vi "APDM Hardware.vi"(7 "Gyro Channel In":T3) -> (2 "GPD Message Channel":T2, 3 "Gyro Status Channel":T4)   [LabVIEW 2019]
uses:
  <extravilib>/ChannelInstances/Messenger-t'Gyro Status Message.ctl'/))Channel.ctl
  Lee Lab/CP FES Walking 2018/Code/Working/LabVIEW/Controls/Messages/Gyro Status Message.ctl
  Lee Lab/CP FES Walking 2018/Code/Working/LabVIEW/Controls/States/Gyro Status States.ctl
  <extravilib>/ChannelInstances/Messenger-t'Acquisition Message.ctl'/))Channel.ctl
  Lee Lab/CP FES Walking 2018/Code/Working/LabVIEW/Controls/Messages/Acquisition Message.ctl
  Lee Lab/CP FES Walking 2018/Code/Working/LabVIEW/Controls/States/Acquisition State.ctl
  <extravilib>/ChannelInstances/Messenger-t'GPD Message.ctl'/))Channel.ctl
  Lee Lab/CP FES Walking 2018/Code/Working/LabVIEW/Controls/Messages/GPD Message.ctl
  Lee Lab/CP FES Walking 2018/Code/Working/LabVIEW/Controls/States/GPD State.ctl
  APDM Data.ctl
  APDM Context Cluster.ctl
  Gyro Status Data.ctl
  <extravilib>/ChannelInstances/Messenger-t'Acquisition Message.ctl'/Read With Abort.vi
  <extravilib>/ChannelInstances/Messenger-t'Gyro Status Message.ctl'/Write With Abort.vi
  <extravilib>/ChannelInstances/Messenger-t'Acquisition Message.ctl'/Write With Abort.vi
  <extravilib>/ChannelInstances/Messenger-t'GPD Message.ctl'/Write With Abort.vi
  <resource>/Channels/Messenger/Read With Abort.vi
  <vilib>/ChannelSupport/Channel Message/Read ID.vi
  <resource>/Channels/Messenger/Write With Abort.vi
  <extravilib>/ChannelInstances/Messenger-t'Gyro Status Message.ctl'/Wrapper.lvclass
  C:/Program Files/National Instruments/LabVIEW 2019/vi.lib/ChannelSupport/Channel Message/Channel Message.lvclass
  <extravilib>/ChannelInstances/Messenger-t'Acquisition Message.ctl'/Wrapper.lvclass
  <extravilib>/ChannelInstances/Messenger-t'GPD Message.ctl'/Wrapper.lvclass
  <resource>/Channels/Messenger/Endpoint.vi
  <extravilib>/ChannelInstances/Messenger-t'Acquisition Message.ctl'/Unwrap.vi
  <extravilib>/ChannelInstances/Messenger-t'Gyro Status Message.ctl'/Wrap.vi
  <extravilib>/ChannelInstances/Messenger-t'Acquisition Message.ctl'/Wrap.vi
  <extravilib>/ChannelInstances/Messenger-t'GPD Message.ctl'/Wrap.vi
  <extravilib>/ChannelInstances/Messenger-t'Acquisition Message.ctl'.lvlib
  <extravilib>/ChannelInstances/Messenger-t'Gyro Status Message.ctl'.lvlib
  <extravilib>/ChannelInstances/Messenger-t'GPD Message.ctl'.lvlib
panel:
  out "Acquisition State":T1
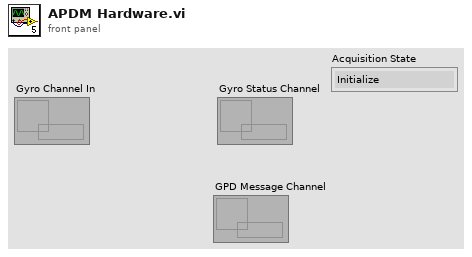
[diagram p1: front panel]
types:
  T1 = typedef "Acquisition State.ctl" = enum16{"Initialize", "Init Hardware", "On", "Off", "Stop"}
  T2 = typedef "Messenger-t'GPD Message.ctl'.lvlib/))Channel.ctl" = refnum<queue>
  T3 = typedef "Messenger-t'Acquisition Message.ctl'.lvlib/))Channel.ctl" = refnum<queue>
  T4 = typedef "Messenger-t'Gyro Status Message.ctl'.lvlib/))Channel.ctl" = refnum<queue>
  T5 = typedef "APDM Data.ctl" = cluster{"Iteration time":u32, "Total elapsed time":u32, "APDM Context":T6}
  T6 = typedef "APDM Context Cluster.ctl" = cluster{"APDM Context ID":u32, "Gyro Mode":string, "Log Data":bool, "Log File":refnum<file>, "Gyro Record Log":refnum<queue>, "Gyro CMD Log":refnum<queue>, "L Opal SN":u32, "R Opal SN":u32, "Access Point ID":u32, "Left Gyro Sim Data":path, "Right Gyro Sim Data":path, "Sampling Rate":dbl, "Gyro Sim Time Array":dbl[], "Missed Gyro Count":dbl}
  T7 = typedef "Acquisition Message.ctl" = cluster{"Acquisition State":T1, "Data":variant}
  T8 = typedef "Gyro Status Data.ctl" = cluster{"Acquisition State":T1, "Data":variant}
  T9 = typedef "Gyro Status Message.ctl" = cluster{"Message":T10, "Data":variant}
  T10 = typedef "Gyro Status States.ctl" = enum16{"Update"}
  T11 = typedef "GPD Message.ctl" = cluster{"GPD State":T12, "Data":variant}
  T12 = typedef "GPD State.ctl" = enum16{"On", "Stop", "Idle", "Initialize", "Update GPD Params", "Reload GPD Params", "Detect Event"}
  T13 = typedef "Gyro Data.ctl" = cluster{"Time":dbl, "Normalization Time":dbl, "Sampling Rate":dbl, "Left Gyro Data":T14, "Right Gyro Data":T14}
  T14 = typedef "Gyro Side Data.ctl" = cluster{"Time":dbl, "Gyro Array Data":dbl[], "Gyro Negation":T15, "Gyro Data":cluster{"Gyro X":dbl, "Gyro Y":dbl, "Gyro Z":dbl}, "Gyro Latency":dbl, "Normalization Time":dbl, "Sampling Rate":dbl}
  T15 = typedef "Gyro Negation.ctl" = bool[]
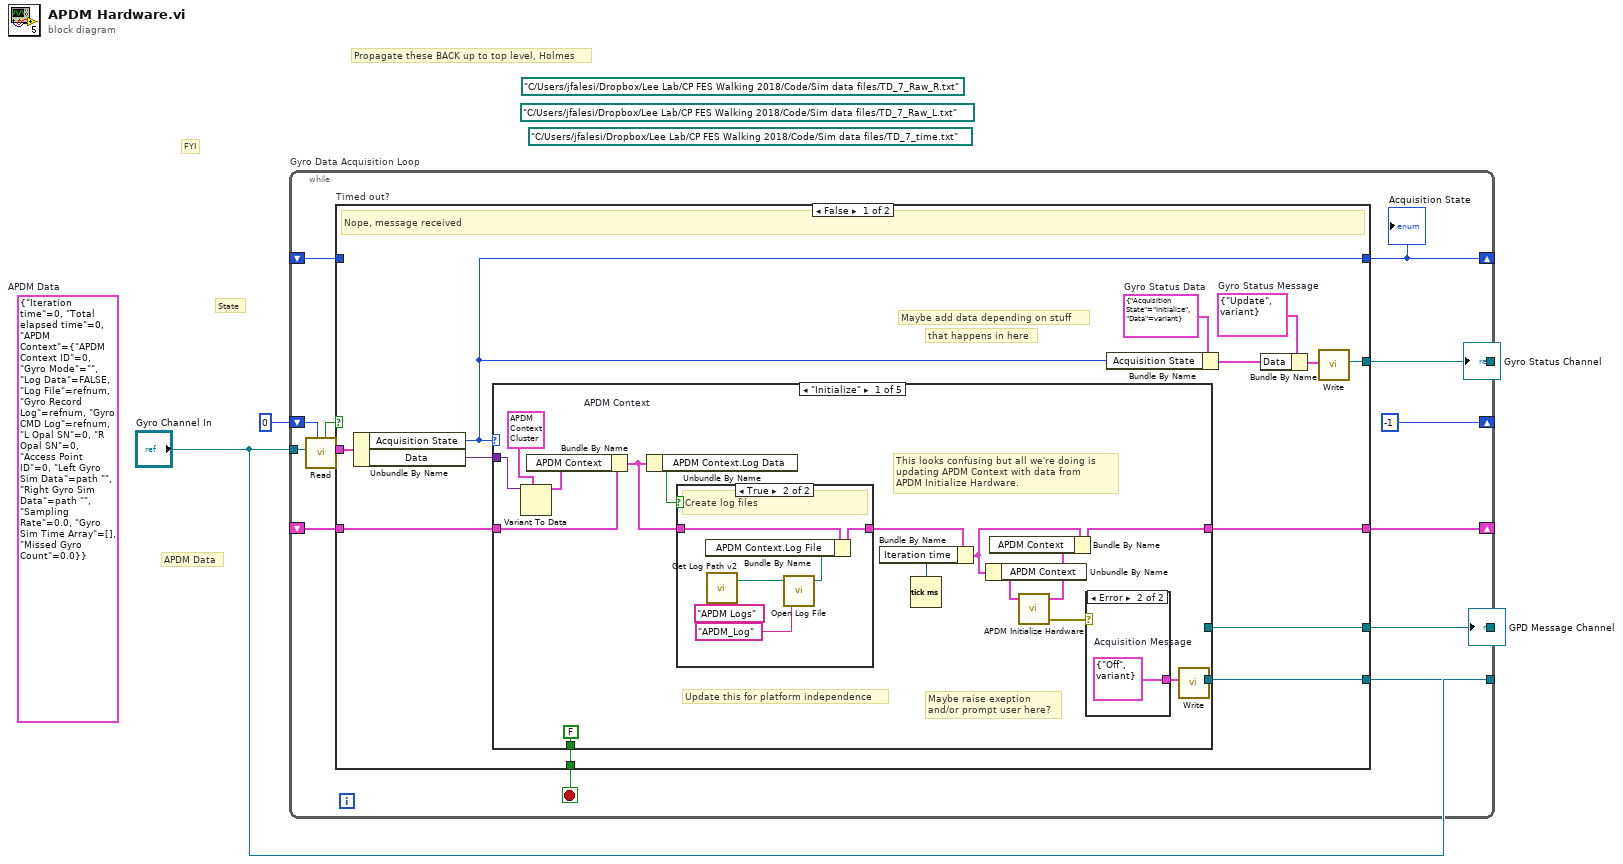
[diagram p0: block diagram]
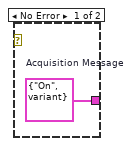
[diagram p3: hidden frame]
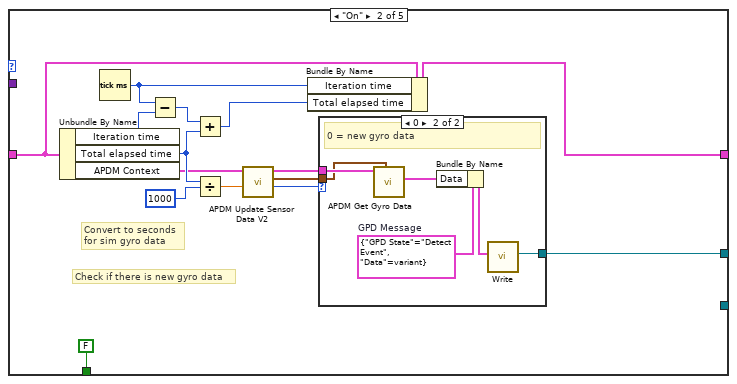
[diagram p4: hidden frame]
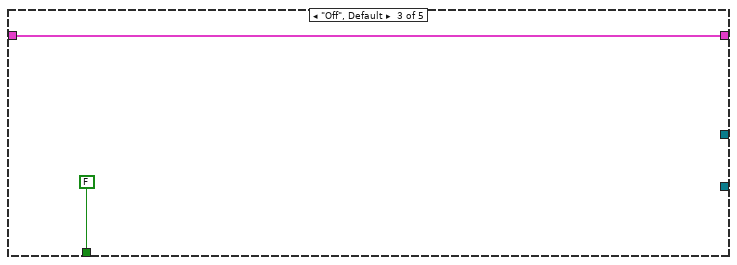
[diagram p6: hidden frame]
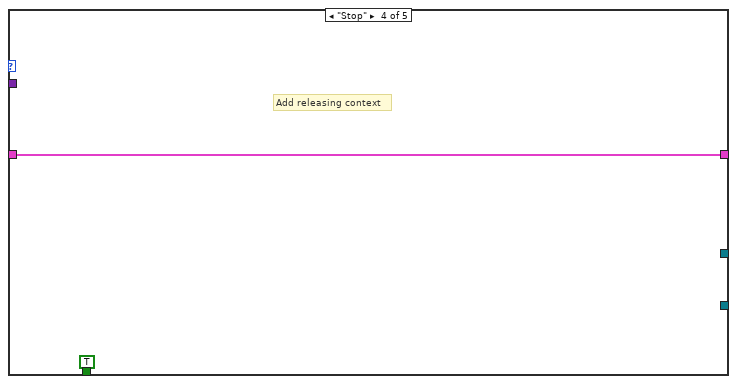
[diagram p7: hidden frame]
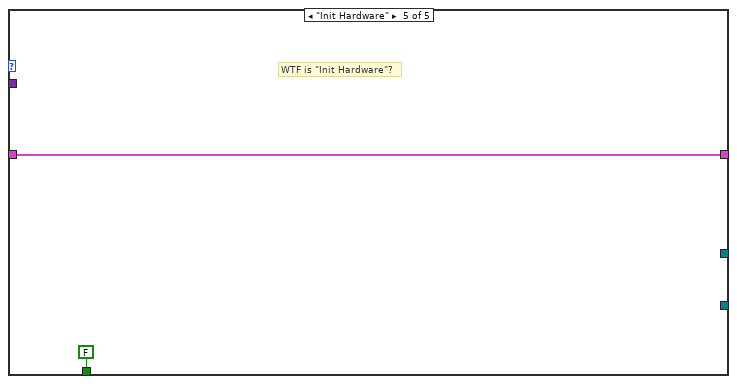
[diagram p8: hidden frame]
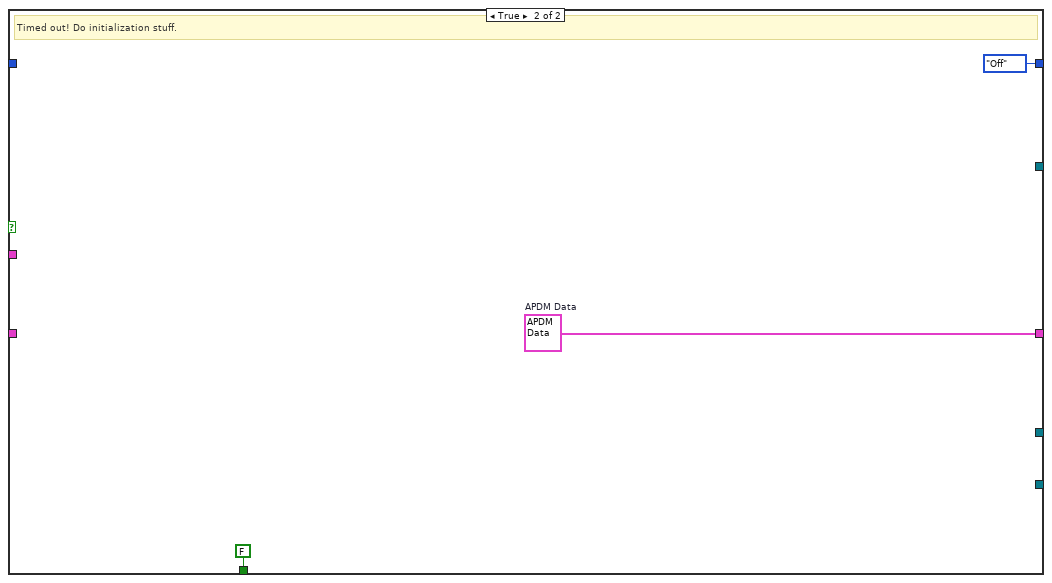
[diagram p9: hidden frame]
diagram:
  (unwired) T5 {"Iteration time"=0, "Total elapsed time"=0, "APDM Context"={"APDM Context ID"=0, "Gyro Mode"="", "Log Data"=FALSE, "Log File"=refnum, "Gyro Record Log"=refnum, "Gyro CMD Log"=refnum, "L Opal SN"=0, "R Opal SN"=0, "Access Point ID"=0, "Left Gyro Sim Data"=path "", "Right Gyro Sim Data"=path "", "Sampling Rate"=0.0, "Gyro Sim Time Array"=[], "Missed Gyro Count"=0.0}}  # APDM Data
  (unwired) path "C:/Users/jfalesi/Dropbox/Lee Lab/CP FES Walking 2018/Code/Sim data files/TD_7_time.txt" ("Gyro Sim Time Data")
  (unwired) path "C:/Users/jfalesi/Dropbox/Lee Lab/CP FES Walking 2018/Code/Sim data files/TD_7_Raw_R.txt" ("Right Gyro Sim Data")
  (unwired) path "C:/Users/jfalesi/Dropbox/Lee Lab/CP FES Walking 2018/Code/Sim data files/TD_7_Raw_L.txt" ("Left Gyro Sim Data")
  # "FYI"
  # "APDM Data"
  # "Propagate these BACK up to top level, Holmes"
  # "State"
  n1 = while "Gyro Data Acquisition Loop" {
    tunnel: "Gyro Channel In" -> [w17]
    tunnel: "Gyro Channel In" -> [w16]
    shift-right: [w5] -> _
    shift-left: _ -> [w6]
    tunnel: [w7] -> w4
    tunnel: [w14] -> w2
    shift-right: [-1 ("timeout in ms (-1)")] -> _
    shift-left: 0 ("timeout in ms (-1)") -> [w12]
    shift-right: [w10] -> _
    shift-left: _ -> [w9]
    stop <- w15 stop-if-true
    n2 = call <extravilib>:"Read.vi"("timeout in ms (-1)"=w12, "channel"=w17) -> ("element"=w11:T7, "timedout?"=w13:bool)  [unwired: 6 in, 2 out]
    n3 = case "Timed out?" shown="False" w13 {
      tunnel: [w30 _] -> w16
      tunnel: [w29 FALSE] -> w15
      tunnel: [w28 _] -> w14
      tunnel: w11 -> [w27 _]
      tunnel: [w24 w85] -> w10
      tunnel: w9 -> [w25 _]
      tunnel: [w21 _] -> w7
      tunnel: w6 -> [_ _]
      tunnel: [w18 Acquisition_State."Off" ("Acquisition State")] -> w5
      frame False {
        w20 = T8 {"Acquisition State"=enum."Initialize", "Data"=variant}  # Gyro Status Data
        w22 = T9 {"Message"=enum."Update", "Data"=variant}  # Gyro Status Message
        # "that happens in here"
        # "Maybe add data depending on stuff"
        # "Nope, message received"
        n4 = Unbundle By Name(w27) -> ("Acquisition State"=w18:T1, "Data"=w26:variant)
        n5 = case shown="\"Initialize\"" w18 {
          tunnel: [w44 _ _ _ _] -> w30
          tunnel: [FALSE FALSE FALSE TRUE FALSE] -> w29
          tunnel: [_ w59 _ _ _] -> w28
          tunnel: w26 -> [w32 _ _ _ _]
          tunnel: w25 -> [w35 w58 w77 w79 w82]
          tunnel: [w36 w57 w77 w79 w82] -> w24
          frame "Initialize" {
            w33 = T6 {"APDM Context ID"=0, "Gyro Mode"="", "Log Data"=FALSE, "Log File"=refnum, "Gyro Record Log"=refnum, "Gyro CMD Log"=refnum, "L Opal SN"=0, "R Opal SN"=0, "Access Point ID"=0, "Left Gyro Sim Data"=path "C:/Users/jfalesi/Desktop/CP FES Walking Code/Original/Ahad Vi/CP Code/Offline data/TD_7_Raw_R.txt", "Right Gyro Sim Data"=path "C:/Users/jfalesi/Desktop/CP FES Walking Code/Original/Ahad Vi/CP Code/Offline data/TD_7_Raw_R.txt", "Sampling Rate"=0.0, "Gyro Sim Time Array"=[], "Missed Gyro Count"=0.0}  # APDM Context
            # "Maybe raise exeption\nand/or prompt user here?"
            # "This looks confusing but all we're doing is \nupdating APDM Context with data from\nAPDM Initialize Hardware."
            # "Update this for platform independence"
            n6 = Variant To Data(type=w33, Variant=w32) -> (data=w31:T6)  [unwired: 1 in, 1 out]
            n7 = Bundle By Name(cluster=w35, "APDM Context"=w31) -> (w34:T5)
            n8 = Unbundle By Name(w34) -> ("APDM Context.Log Data"=w42:bool)
            n9 = case shown="True" w42 {
              tunnel: w34 -> [w47 w50]
              tunnel: [w47 w48] -> w40
              frame False {
              }
              frame True {
                # "Create log files"
                n10 = call "Get Log Path v2.vi"("Log Dir Name"="APDM Logs") -> ("Log Path"=w53:path)  [unwired: 2 in]
                n11 = call "Open Log File .vi"("File Name Snippet"="APDM_Log", "Log Path"=w53) -> ("Byte Stream File out"=w49:refnum<file>)  [unwired: 2 in, 1 out]
                n12 = Bundle By Name(cluster=w50, "APDM Context.Log File"=w49) -> (w48:T5)
              }
            }
            n13 = Tick Count (ms) ("Elapsed Time (ms)")() -> (millisecond timer value=w41:u32)
            n14 = Bundle By Name(cluster=w40, "Iteration time"=w41) -> (w37:T5)
            n15 = Unbundle By Name(w37) -> ("APDM Context"=w39:T6)
            n16 = call "APDM Initialize Hardware.vi"("APDM Context in"=w39) -> ("error out"=w46:errorcluster, "APDM Context out"=w38:T6)  [unwired: 3 in]
            n17 = Bundle By Name(cluster=w37, "APDM Context"=w38) -> (w36:T5)
            n18 = case shown="Error" w46 {
              tunnel: [w54 w55] -> w45
              frame No Error {
                w54 = T7 {"Acquisition State"=enum."On", "Data"=variant}  # Acquisition Message
              }
              frame Error {
                w55 = T7 {"Acquisition State"=enum."Off", "Data"=variant}  # Acquisition Message
              }
            }
            n19 = call <extravilib>:"Write.vi"("element"=w45) -> ("channel"=w44:T3)  [unwired: 8 in, 2 out]
          }
          frame "On" {
            # "Convert to seconds\nfor sim gyro data"
            # "Check if there is new gyro data"
            n20 = Unbundle By Name(w58) -> ("Iteration time"=w70:u32, "Total elapsed time"=w66:u32, "APDM Context"=w56:T6)
            n21 = Tick Count (ms) ("Elapsed Time (ms)")() -> (millisecond timer value=w68:u32)
            n22 = Subtract(x=w68, y=w70) -> (x-y=w69:u32)
            n23 = Add(x=w69, y=w66) -> (x+y=w67:u32)
            n24 = Divide(x=w66, y=u32 1000) -> (x/y=w64:dbl)
            n25 = call "APDM Update Sensor Data V2.vi"("Elapsed Time (for sim gyro)"=w64, "APDM Context"=w56) -> ("Result"=w63:u32, "Gyro Cluster Thingy"=w61:cluster{i32, dbl}, "APDM Context Out"=w62:T6)  [unwired: 4 in, 2 out]
            n26 = Bundle By Name(cluster=w58, "Iteration time"=w68, "Total elapsed time"=w67) -> (w57:T5)
            n27 = case shown="0" w63 {
              tunnel: w62 -> [_ w76]
              tunnel: w61 -> [_ w75]
              tunnel: [_ w72] -> w59
              frame 4, Default {
                # "4 = no new data"
              }
              frame 0 {
                w74 = T11 {"GPD State"=enum."Detect Event", "Data"=variant}  # GPD Message
                # "0 = new gyro data"
                n28 = call "APDM Get Gyro Data.vi"("Sim Gyro Cluster"=w75, "APDM Context"=w76) -> ("Gyro Data"=w71:T13)  [unwired: 4 in, 3 out]
                n29 = Bundle By Name(cluster=w74, "Data"=w71) -> (w73:T11)
                n30 = call <extravilib>:"Write.vi"("element"=w73) -> ("channel"=w72:T2)  [unwired: 8 in, 2 out]
              }
            }
          }
          frame "Off", Default {
          }
          frame "Stop" {
            # "Add releasing context"
          }
          frame "Init Hardware" {
            # "WTF is \"Init Hardware\"?"
          }
        }
        n31 = Bundle By Name(cluster=w20, "Acquisition State"=w18) -> (w19:T8)
        n32 = Bundle By Name(cluster=w22, "Data"=w19) -> (w23:T9)
        n33 = call <extravilib>:"Write.vi"("element"=w23) -> ("channel"=w21:T4)  [unwired: 8 in, 2 out]
      }
      frame True {
        w85 = T5 {"Iteration time"=0, "Total elapsed time"=0, "APDM Context"={"APDM Context ID"=0, "Gyro Mode"="", "Log Data"=FALSE, "Log File"=refnum, "Gyro Record Log"=refnum, "Gyro CMD Log"=refnum, "L Opal SN"=0, "R Opal SN"=0, "Access Point ID"=0, "Left Gyro Sim Data"=path "", "Right Gyro Sim Data"=path "", "Sampling Rate"=0.0, "Gyro Sim Time Array"=[], "Missed Gyro Count"=0.0}}  # APDM Data
        # "Timed out! Do initialization stuff."
      }
    }
    "Acquisition State" <- w5
  }
  "Gyro Status Channel" <- w4
  "GPD Message Channel" <- w2
